vi "VISCOCITY 2.vi"() -> ()   [LabVIEW 2014]
panel:
  out "Numeric Control 2":dbl
  out "x-y":dbl
  out "Numeric Control":dbl
  out "x .or. y?":bool
  out ".not. x?":bool
  out "x = y?":bool
  in  "Tab Control":T1(tab)
  in  "?":dbl(slide)=29.292929292929294 scale=0.0..100.0
  out "?":bool
  in  "?":T2(ring)
  in  "STOP":bool
  out "?":u8(slide) scale=0.0..115.0
  out "Ve":u8(slide) scale=0.0..400.0
  out "?":dbl format="%#_4g"
  out "?":dbl format="%#_4g"
  out "?":u8(slide) scale=0.0..50.0
  out "?":bool
  out "Temperature Vs Time":cluster{"Y":dbl[], "Y":dbl[]}[](graph)
  out "1 2":string[][](table)
  out "?":dbl format="%#_4g"
  out "Ve 2":u8(slide) scale=0.0..50.0
  out "Ve 3":u8(slide) scale=0.0..145.0
  # "Manipal Institute of Technology  \n        Dept of Instrumentation and Control Engineering\n                                 V Sem (Instrumentation Lab)"
  # "VIRTUAL LABS"
  # "VIRTUAL LABS"
  # "Measurement of Viscosity\n\nAim:\n\n To measure the Kinematic viscosity of the oil sample.\n\nApparatus required:\n\n\tSaybolt Viscosity Equipment.\n\tThermometer.\n\t Stop watch.\n\nInstructions:\n\n\tFirst use the Saybolt Viscometer to investigate the possible dependence of the viscosity of an SAE 10w-30-oil sample, at room temperature, on the rate of applied shear.\n\tNext you are required to measure the viscosity of the oil at 5 different temperatures above \"Room Temperature\" each at a ?T higher than the preceding one.\n\t Temperatures should range from \"Room Temperature\" to a temperature like 90°C or 95°C near the boiling point of water.\n\tChoose a convenient ?T in degrees C to accomplish this which will allow you to calculate the required set-point temperatures need by the constant temperature bath controller.\n\tOnce the tests with the oil have been completed set the next desired temperature and turn on the controller.\n\tThe oil level will then begin to fall. Use the electric timer to measure the elapsed time it takes the oil level to fall from point C to point E.\n\tHere it is the time required to fill a 60 ml flask located below the viscometer without that runs out of a large reservoir through a capillary tube. You will find this viscometer filled with oil to the proper level.\n\tTo start the flow, simply remove the cork at the bottom of the reservoir. At this point start the timer and stop it when the level of the oil at the flask reaches the indicator line.\n\tImmediately replace the cork so as to stop the flow and prevent the remaining oil in the reservoir from running out.\n\tUnderstand that while this is a simple process it can also get messy. Be careful and place the collecting flask under the viscometer so that the oil falls into the flask and does not hit the glass.\n\tMake sure you wipe off your hands before picking up the flask and pouring its contents back into the reservoir If the oil level in the reservoir is low add a little new oil before taking the next data value.\n\tInvert the first collection flask on a paper towel and allow it to drain before using it again.\n\nCalculations:\n\n\n\t                                                   For t < 100s                                 v=0.00226t-1.95/t\n\n\n                                       \tFor t > 100s                                 v=0.00220t-1.35/t"
  # "EXPERIMENT NO.1"
  # "Select Temperature"
  # "Time"
  # "Temperature (deg)"
  # "Time (Sec)"
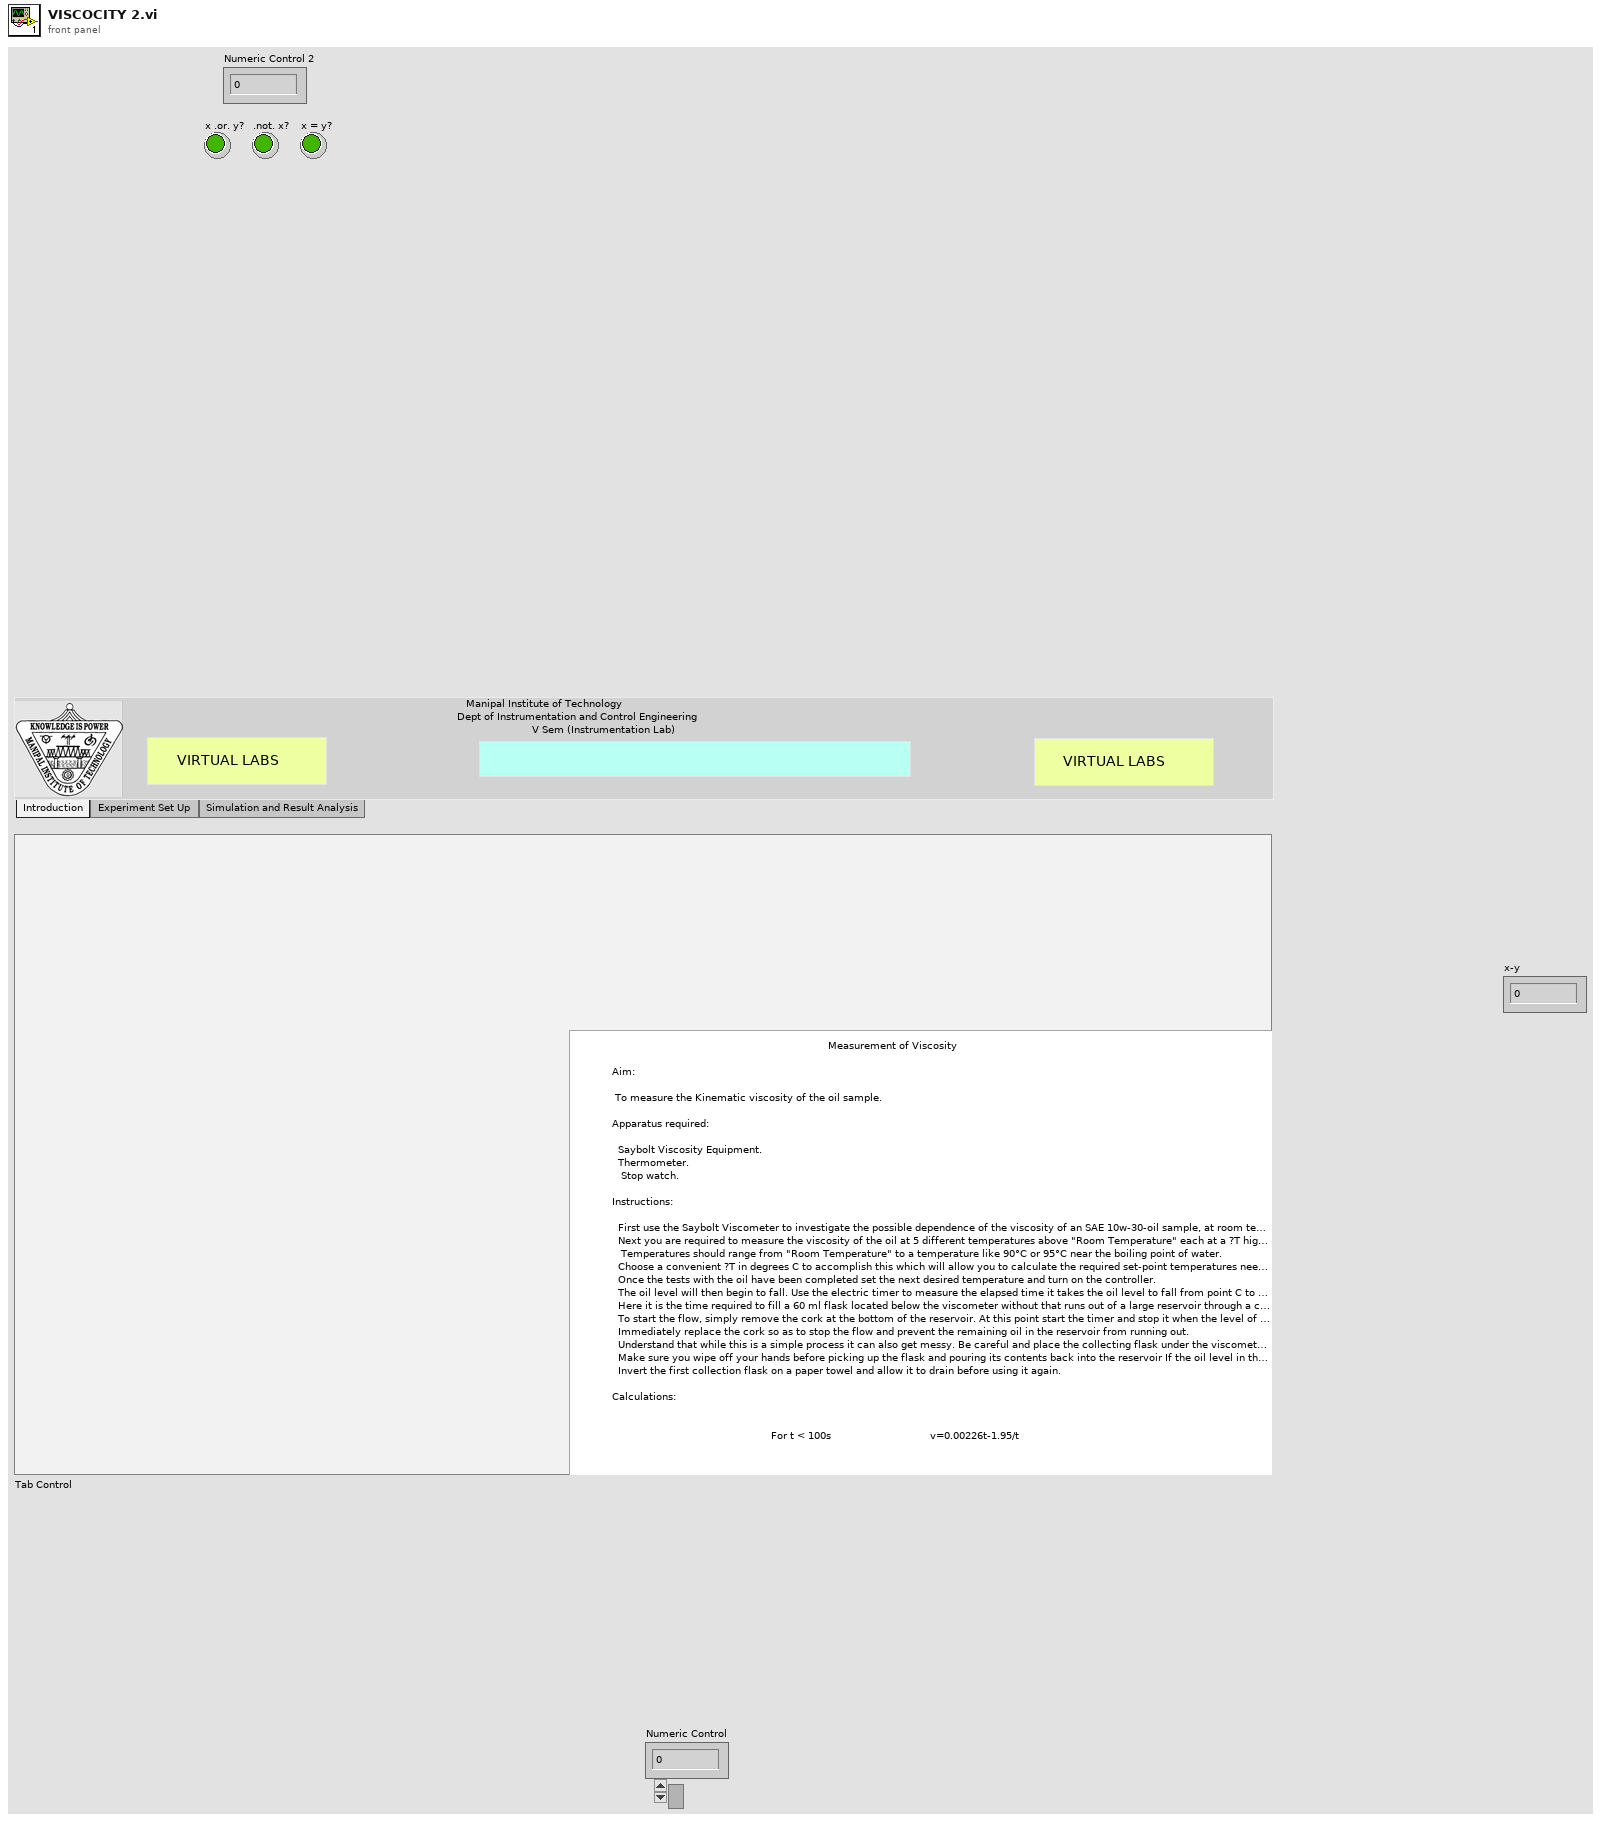
[diagram p1: front panel]
types:
  T1 = enum32{"Introduction", "Experiment Set Up ", "Simulation and Result Analysis"}
  T2 = enum16{"30", "35", "42", "50", "60", "72", "90", ""}
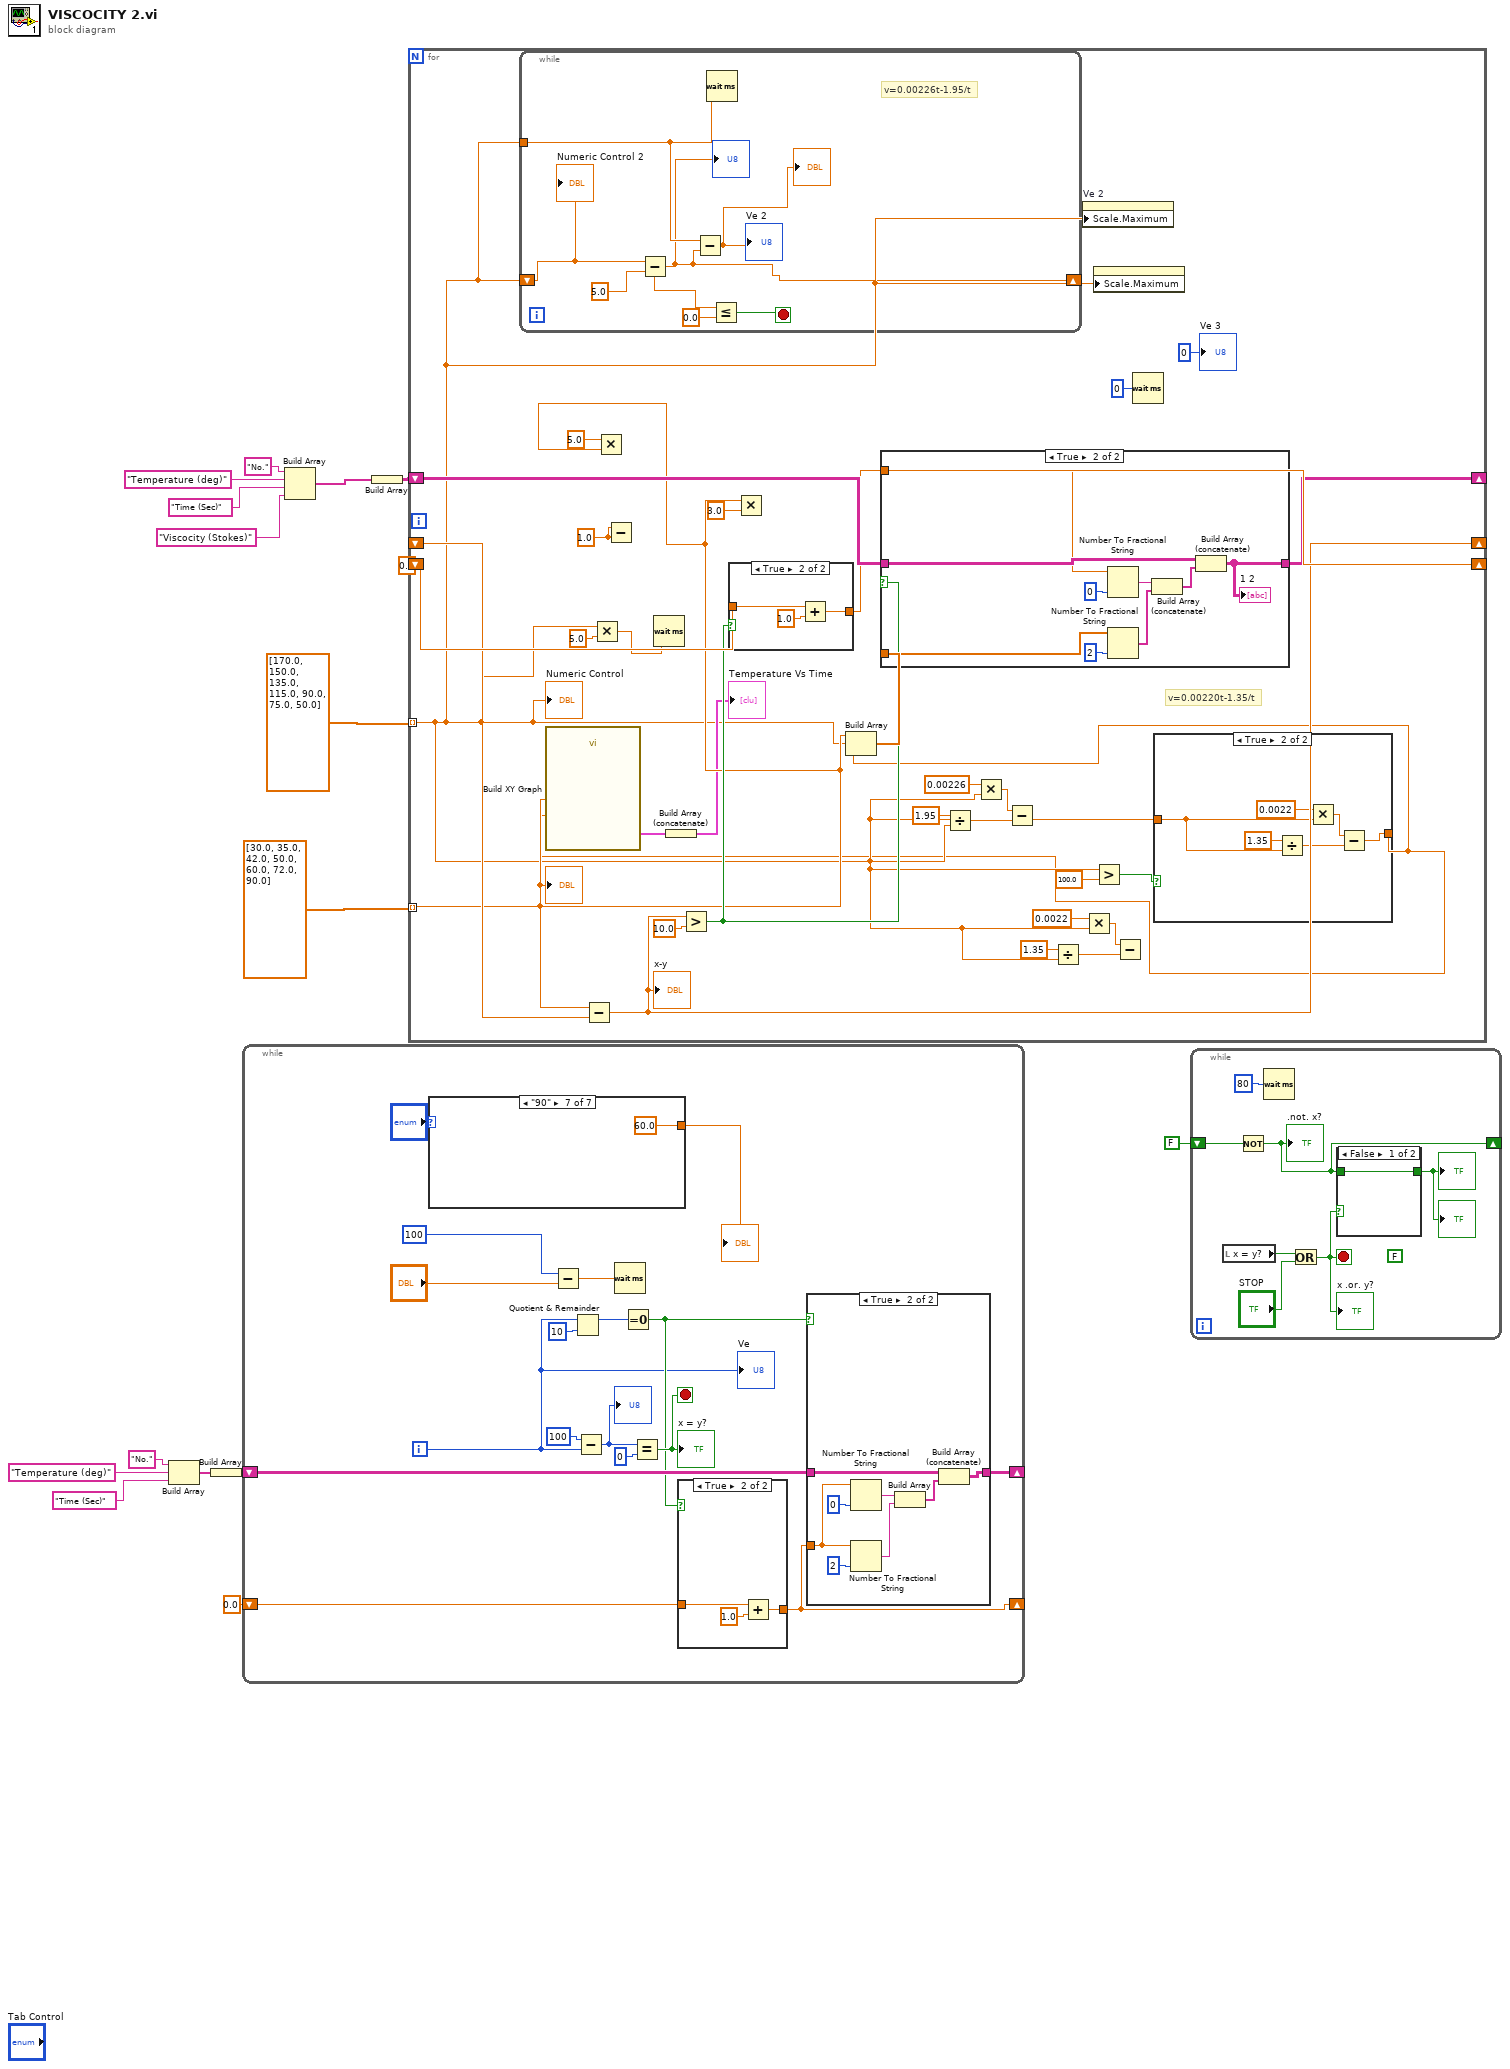
[diagram p0: block diagram]
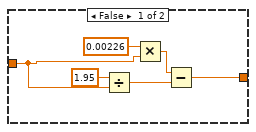
[diagram p2: hidden frame]
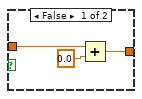
[diagram p4: hidden frame]
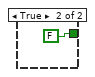
[diagram p5: hidden frame]
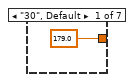
[diagram p6: hidden frame]
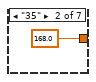
[diagram p7: hidden frame]
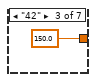
[diagram p8: hidden frame]
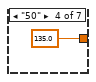
[diagram p9: hidden frame]
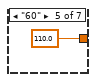
[diagram p10: hidden frame]
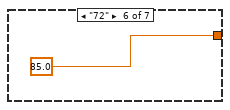
[diagram p11: hidden frame]
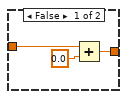
[diagram p12: hidden frame]
diagram:
  n1 = Build Array("No." ("element"), "Temperature (deg)" ("element"), "Time (Sec)") -> (w14:string[])
  n2 = Build Array(w14) -> (w11:string[][])
  n3 = while {
    shift-right: [w30] -> _
    shift-left: w11 -> [w29]
    shift-right: [w25] -> _
    shift-left: 0.0 -> [w26]
    i -> [w18]
    stop <- w31 stop-if-true
    n4 = case shown="\"90\"" "?" {
      tunnel: [179.0 168.0 150.0 135.0 110.0 85.0 60.0] -> w17
      frame "30", Default {
      }
      frame "35" {
      }
      frame "42" {
      }
      frame "50" {
      }
      frame "60" {
      }
      frame "72" {
      }
      frame "90" {
      }
    }
    "?" <- w17
    n5 = Subtract(x=u32 100 ("milliseconds to wait"), y="?") -> (x-y=w20:dbl)
    n6 = Quotient & Remainder(x=w18, y=10) -> (x-y*floor(x/y)=w28:i32)  [unwired: 1 out]
    n7 = Subtract(x=100, y=w18) -> (x-y=w23:i32)
    "?" <- w23
    n8 = Wait (ms)(milliseconds to wait=w20) -> ()  [unwired: 1 out]
    n9 = Equal To 0?(x=w28) -> (x = 0?=w24:bool)
    n10 = Equal?(x=w23, y=0) -> (x = y?=w31:bool)
    "x = y?" <- w31
    n11 = case shown="True" w24 {
      tunnel: w26 -> [w42 w46]
      tunnel: [w41 w45] -> w25
      frame False {
        n12 = Add(x=w42, y=0.0) -> (x+y=w41:dbl)
      }
      frame True {
        n13 = Add(x=w46, y=1.0) -> (x+y=w45:dbl)
      }
    }
    n14 = case shown="True" w24 {
      tunnel: w29 -> [w47 w50]
      tunnel: [w47 w49] -> w30
      tunnel: w25 -> [_ w48]
      frame False {
      }
      frame True {
        n15 = Number To Fractional String(number=w48, precision (6)=i16 0) -> (F-format string=w53:string)  [unwired: 2 in]
        n16 = Number To Fractional String(number=w48, precision (6)=i16 2) -> (F-format string=w52:string)  [unwired: 2 in]
        n17 = Build Array(w53, w52) -> (w51:string[])
        n18 = Build Array (concatenate)(w50, w51) -> (w49:string[][])
      }
    }
    "Ve" <- w18
  }
  n19 = Build Array("No." ("element"), "Temperature (deg)" ("element"), "Time (Sec)", "Viscocity (Stokes)") -> (w5:string[])
  n20 = Build Array(w5) -> (w3:string[][])
  n21 = for {
    tunnel: dbl[] [170.0, 150.0, 135.0, 115.0, 90.0, 75.0, 50.0] -> [w57] mode=indexing
    tunnel: dbl[] [30.0, 35.0, 42.0, 50.0, 60.0, 72.0, 90.0] -> [w73] mode=indexing
    shift-right: [w76] -> _
    shift-left: w3 -> [w84]
    shift-right: [w82] -> _
    shift-left: 0.0 -> [w83]
    shift-right: [w79] -> _
    shift-left: _ -> [w80]
    w72 = 1.0 ("y")
    # "v=0.00220t-1.35/t"
    n22 = while {
      shift-right: [w100] -> _
      shift-left: w57 -> [w105]
      tunnel: w57 -> [w101]
      stop <- w103 stop-if-true
      # "v=0.00226t-1.95/t"
      n23 = Subtract(x=w105, y=5.0) -> (x-y=w100:dbl)
      "?" <- w100
      n24 = Subtract(x=w101, y=w100) -> (x-y=→"Ve 2" →"?":dbl)
      n25 = Wait (ms)(milliseconds to wait=w101) -> ()  [unwired: 1 out]
      n26 = Less Or Equal?(x=w100, y=0.0) -> (x <= y?=w103:bool)
      "Numeric Control 2" <- w105
    }
    n27 = Subtract(x=w73, y=w80) -> (x-y=w79:dbl)
    "x-y" <- w79
    n28 = Multiply(x=w57, y=5.0) -> (x*y=w70:dbl)
    n29 = Multiply(x=5.0, y=w73) -> ()  [unwired: 1 out]
    n30 = Subtract(x=w72, y=w72) -> ()  [unwired: 1 out]
    n31 = Wait (ms)(milliseconds to wait=w70) -> ()  [unwired: 1 out]
    n32 = Greater?(x=w79, y=10.0) -> (0:w77:bool)
    n33 = case shown="True" w77 {
      tunnel: w83 -> [w117 w121]
      tunnel: [w116 w120] -> w82
      frame False {
        n34 = Add(x=w117, y=0.0) -> (x+y=w116:dbl)
      }
      frame True {
        n35 = Add(x=w121, y=1.0) -> (x+y=w120:dbl)
      }
    }
    n36 = Multiply(x=w73, y=3.0) -> ()  [unwired: 1 out]
    n37 = Divide(x=1.95, y=w57) -> (x/y=w66:dbl)
    n38 = Multiply(x=0.00226, y=w57) -> (x*y=w64:dbl)
    n39 = Subtract(x=w64, y=w66) -> ()  [unwired: 1 out]
    n40 = Divide(x=1.35, y=w57) -> (x/y=w61:dbl)
    n41 = property on="Ve 2" class="Slide (strict)"("Scale.Maximum"=w57) -> ()  [unwired: 2 in, 2 out]
    n42 = Multiply(x=0.0022, y=w57) -> (x*y=w63:dbl)
    n43 = property class="Slide (strict)"("Scale.Maximum"=w57) -> ()  [unwired: 2 in, 2 out]
    n44 = Greater?(x=w57, y=100.0) -> (0:w58:bool)
    n45 = Subtract(x=w63, y=w61) -> ()  [unwired: 1 out]
    n46 = Wait (ms)(milliseconds to wait=u32 0) -> ()  [unwired: 1 out]
    n47 = case shown="True" w58 {
      tunnel: w57 -> [w88 w94]
      tunnel: [w87 w93] -> w56
      frame False {
        n48 = Divide(x=1.95, y=w88) -> (x/y=w90:dbl)
        n49 = Multiply(x=0.00226, y=w88) -> (x*y=w92:dbl)
        n50 = Subtract(x=w92, y=w90) -> (x-y=w87:dbl)
      }
      frame True {
        n51 = Divide(x=1.35, y=w94) -> (x/y=w97:dbl)
        n52 = Multiply(x=0.0022, y=w94) -> (x*y=w95:dbl)
        n53 = Subtract(x=w95, y=w97) -> (x-y=w93:dbl)
      }
    }
    n54 = call "Build XY Graph"("Y Input"=w56, "X Input"=w73) -> ("XY Graph"=w86:cluster{"Y":dbl[], "Y":dbl[]}[])  [unwired: 3 in, 6 out]
    n55 = Build Array (concatenate)(w86) -> (→"Temperature Vs Time":cluster{"Y":dbl[], "Y":dbl[]}[])
    n56 = Build Array(w73, w57, w56) -> (w81:dbl[])
    n57 = case shown="True" w77 {
      tunnel: w84 -> [w106 w110]
      tunnel: [w106 w109] -> w76
      tunnel: w82 -> [_ w108]
      tunnel: w81 -> [_ w107]
      frame False {
      }
      frame True {
        n58 = Number To Fractional String(number=w108, precision (6)=i16 0) -> (F-format string=w113:string)  [unwired: 2 in]
        n59 = Number To Fractional String(number=w107, precision (6)=i16 2) -> (F-format string=w112:string[])  [unwired: 2 in]
        n60 = Build Array (concatenate)(w113, w112) -> (w111:string[])
        n61 = Build Array (concatenate)(w110, w111) -> (w109:string[][])
        "1 2" <- w109
      }
    }
    "Numeric Control" <- w57
    "?" <- w73
    "Ve 3" <- u8 0 ("Ve 3")
  }
  n62 = while {
    shift-right: [w124] -> _
    shift-left: FALSE -> [w128]
    stop <- w125 stop-if-true
    (unwired) FALSE
    n63 = local read "x = y?"() -> (w126:bool)
    n64 = Not(x=w128) -> (.not. x?=w124:bool)
    ".not. x?" <- w124
    n65 = Wait (ms)(milliseconds to wait=u32 80) -> ()  [unwired: 1 out]
    n66 = Or(x=w126, y="STOP") -> (x .or. y?=w125:bool)
    "x .or. y?" <- w125
    n67 = case shown="False" w125 {
      tunnel: [w129 FALSE] -> w122
      tunnel: w124 -> [w129 _]
      frame False {
      }
      frame True {
      }
    }
    "?" <- w122
    "?" <- w122
  }
